vi "Set AO anti-aliasingh PXI.vi"(1 "scanrate (Hz)":dbl format="%.2f") -> (0 "anti-aliasing frequency":dbl format="%.2f")   [LabVIEW 2015]
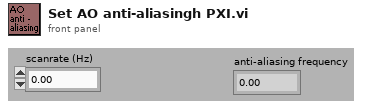
[diagram p1: front panel]
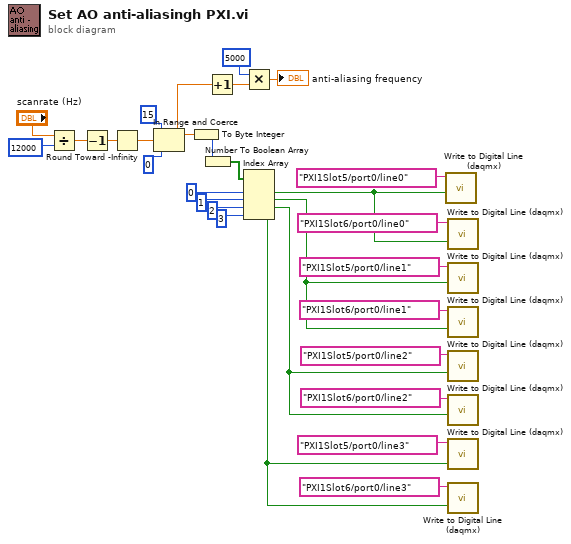
[diagram p0: block diagram]
diagram:
  n1 = Divide(x="scanrate (Hz)", y=12000) -> (x/y=w27:dbl)
  n2 = Decrement(x=w27) -> (x-1=w14:dbl)
  n3 = Round Toward -Infinity(1:w14) -> (0:w13:dbl)
  n4 = In Range and Coerce(upper limit=15, x=w13, lower limit=0) -> (coerced(x)=w20:dbl)  [unwired: 1 out]
  n5 = To Byte Integer(number=w20) -> (8bit integer=w21:i8)
  n6 = Number To Boolean Array(number=w21) -> (Boolean array=w19:bool[])
  n7 = Increment(x=w20) -> (x+1=w24:dbl)
  n8 = Multiply(x=5000, y=w24) -> (x*y=→"anti-aliasing frequency":dbl)
  n9 = Index Array(array=w19, index #1=0, index #2=1, index #3=2, index #4=3) -> (element #1=w18:bool, element #2=w17:bool, element #3=w16:bool, element #4=w15:bool)
  n10 = call "Write to Digital Line (daqmx).vi"("Line State"=w18, "Line"=tag "PXI1Slot5/port0/line0" ("Lines 2")) -> ()  [unwired: 5 in, 1 out]
  n11 = call "Write to Digital Line (daqmx).vi"("Line State"=w18, "Line"=tag "PXI1Slot6/port0/line0" ("Lines 2")) -> ()  [unwired: 5 in, 1 out]
  n12 = call "Write to Digital Line (daqmx).vi"("Line State"=w17, "Line"=tag "PXI1Slot5/port0/line1" ("Lines 2")) -> ()  [unwired: 5 in, 1 out]
  n13 = call "Write to Digital Line (daqmx).vi"("Line State"=w17, "Line"=tag "PXI1Slot6/port0/line1" ("Lines 2")) -> ()  [unwired: 5 in, 1 out]
  n14 = call "Write to Digital Line (daqmx).vi"("Line State"=w16, "Line"=tag "PXI1Slot5/port0/line2" ("Lines 2")) -> ()  [unwired: 5 in, 1 out]
  n15 = call "Write to Digital Line (daqmx).vi"("Line State"=w16, "Line"=tag "PXI1Slot6/port0/line2" ("Lines 2")) -> ()  [unwired: 5 in, 1 out]
  n16 = call "Write to Digital Line (daqmx).vi"("Line State"=w15, "Line"=tag "PXI1Slot5/port0/line3" ("Lines 2")) -> ()  [unwired: 5 in, 1 out]
  n17 = call "Write to Digital Line (daqmx).vi"("Line State"=w15, "Line"=tag "PXI1Slot6/port0/line3" ("Lines 2")) -> ()  [unwired: 5 in, 1 out]
